vi "ConditionalSigned32.vi"(1 "Value in":i32) -> (0 "Stop?":bool)   [LabVIEW 2020]
doc: "Displays the value of the 32-bit signed integer numeric control and allows conditional breakpoints."
panel:
  in  "Tab Control":enum32{"Data   ", "Condition      "}(tab)
  out "Value":i32
  in  "Ls":i32
  in  "Gr":i32
  in  "Eq":i32
  in  "Ls":bool
  in  "Gr":bool
  in  "Eq":bool
  # "Pause if any of the following:"
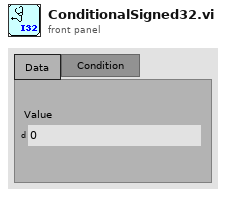
[diagram p1: front panel]
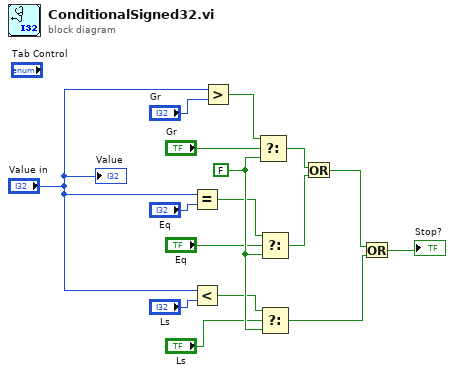
[diagram p0: block diagram]
diagram:
  w12 = FALSE ("f")
  n1 = Equal?(x="Value in", y="Eq") -> (x = y?=w9:bool)
  n2 = Less?(x="Value in", y="Ls") -> (x < y?=w2:bool)
  n3 = Greater?(x="Value in", y="Gr") -> (0:w13:bool)
  n4 = Select(t=w13, s="Gr", f=w12) -> (s? t:f=w6:bool)
  n5 = Select(t=w9, s="Eq", f=w12) -> (s? t:f=w5:bool)
  n6 = Select(t=w2, s="Ls", f=w12) -> (s? t:f=w3:bool)
  n7 = Or(x=w6, y=w5) -> (x .or. y?=w4:bool)
  n8 = Or(x=w4, y=w3) -> (x .or. y?=→"Stop?":bool)
  "Value" <- "Value in"
